vi "Start_DAQ.vi"(7 "platform":u16(ring) items=["Mac", "PC"], 8 "error in (no error)":errorcluster, 9 "Command_Queue_in":T2, 10 "Command_message_in":T1, 11 "DAQ in":refnum<vi>) -> (0 "error out":errorcluster, 3 "Command_message_out":T1)   [LabVIEW 2021]
uses:
  Command_Queue.ctl
  Command_Message.ctl
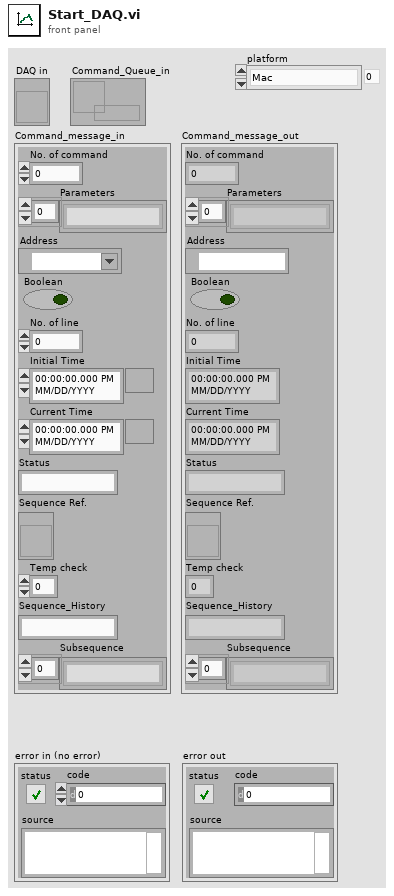
[diagram p1: front panel]
types:
  T1 = typedef "Command_Message.ctl" = cluster{"No. of command":i32, "Parameters":string[], "Address":refnum<visa-resource-name>, "Boolean":bool, "No. of line":i32, "Initial Time":timestamp, "Current Time":timestamp, "Status":string, "Sequence Ref.":refnum<vi>, "Temp check":i32, "Sequence_History":string, "Subsequence":string[]}
  T2 = typedef "Command_Queue.ctl" = refnum<queue>
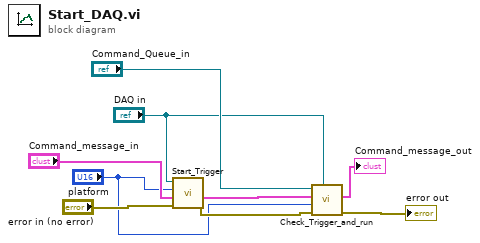
[diagram p0: block diagram]
diagram:
  n1 = call "Start_Trigger.vi"("error in (no error)"="error in (no error)", "Command_Message_in"="Command_message_in", "platform"="platform", "DAQ_VI"="DAQ in") -> ("error out"=w7:errorcluster, "Command_Message_out"=w6:T1)  [unwired: 6 in]
  n2 = call "Check_Trigger_and_run.vi"("DAQ_VI"="DAQ in", "error in (no error)"=w7, "platform"="platform", "Command_Message_in"=w6, "Command_queue_in"="Command_Queue_in") -> ("error out"=→"error out":errorcluster, "Command_Message_out"=→"Command_message_out":T1)  [unwired: 5 in]
